vi "MessageName.vi"() -> (2 "MessageName":string)   [LabVIEW 2020, in "CmdDigital.lvlib"]
uses:
  CmdDigital.lvlib
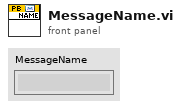
[diagram p1: front panel]
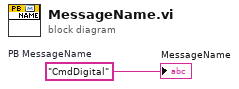
[diagram p0: block diagram]
diagram:
  w1 = "CmdDigital"  # PB MessageName
  "MessageName" <- w1
